vi "worksheet gridlines.vi"(8 "error in (no error)":errorcluster, 10 "option":u8, 11 "worksheet":u32) -> (0 "error out":errorcluster)   [LabVIEW 8.6]
doc: "void worksheet_gridlines(lxw_worksheet worksheet, uint8_t option);"
uses:
  pending_lvxlsxwriter/xlsxwriter.dll
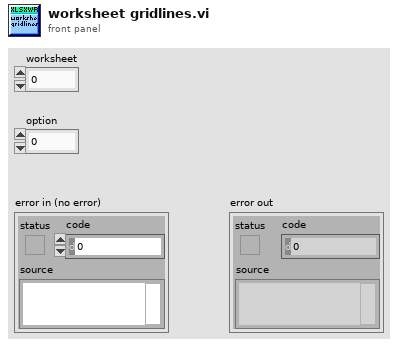
[diagram p1: front panel]
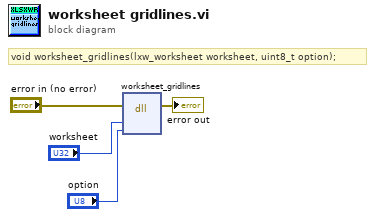
[diagram p0: block diagram]
diagram:
  # "void worksheet_gridlines(lxw_worksheet worksheet, uint8_t option);"
  n1 = dll-call lib="C:/Users/WDAGUtilityAccount/Desktop/pending_lvxlsxwriter/xlsxwriter.*" fn="worksheet_gridlines"(error in="error in (no error)", "worksheet"="worksheet", "option"="option") -> (error out=→"error out":errorcluster)  [unwired: 5 in, 1 out]
